vi "UTL_Generar Reporte.vi"(8 "Error in":errorcluster, 10 "Data":dbl[][](array[numeric]), 11 "Results Path":path) -> (0 "Error out":errorcluster, 3 "Tabla de Datos":string[][](array[string]))   [LabVIEW 2019]
uses:
  Variable global de carga.vi
  <vilib>/Utility/file.llb/Read Delimited Spreadsheet (string).vi
  <vilib>/Utility/file.llb/Write Delimited Spreadsheet (string).vi
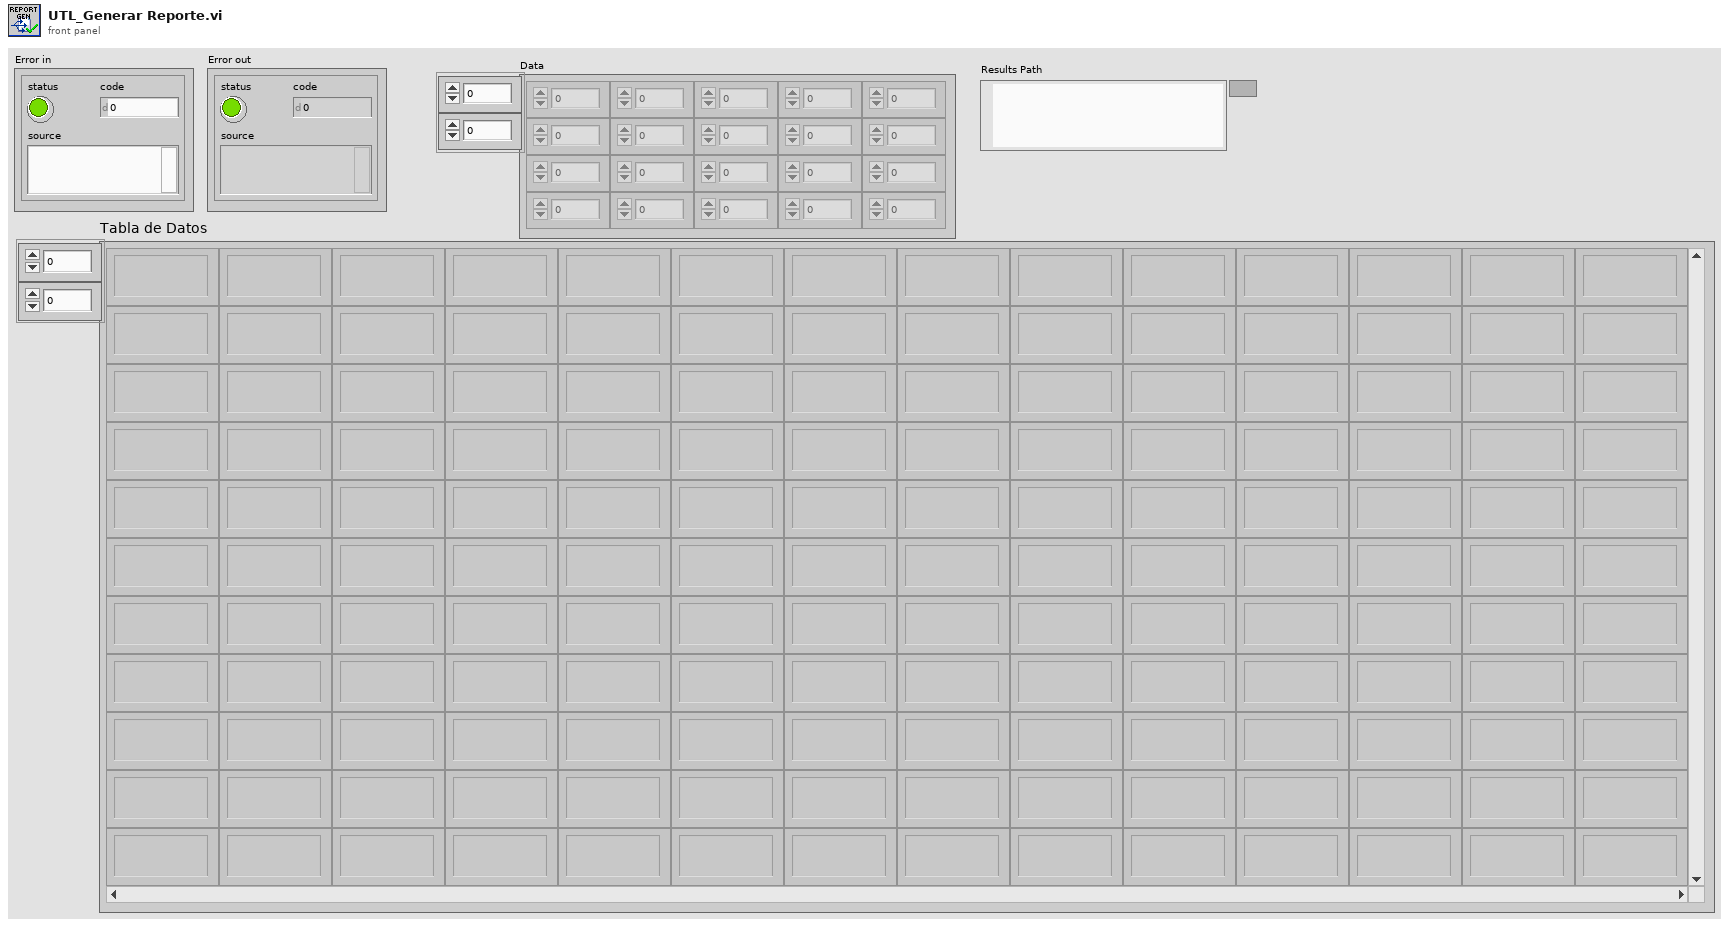
[diagram p1: front panel]
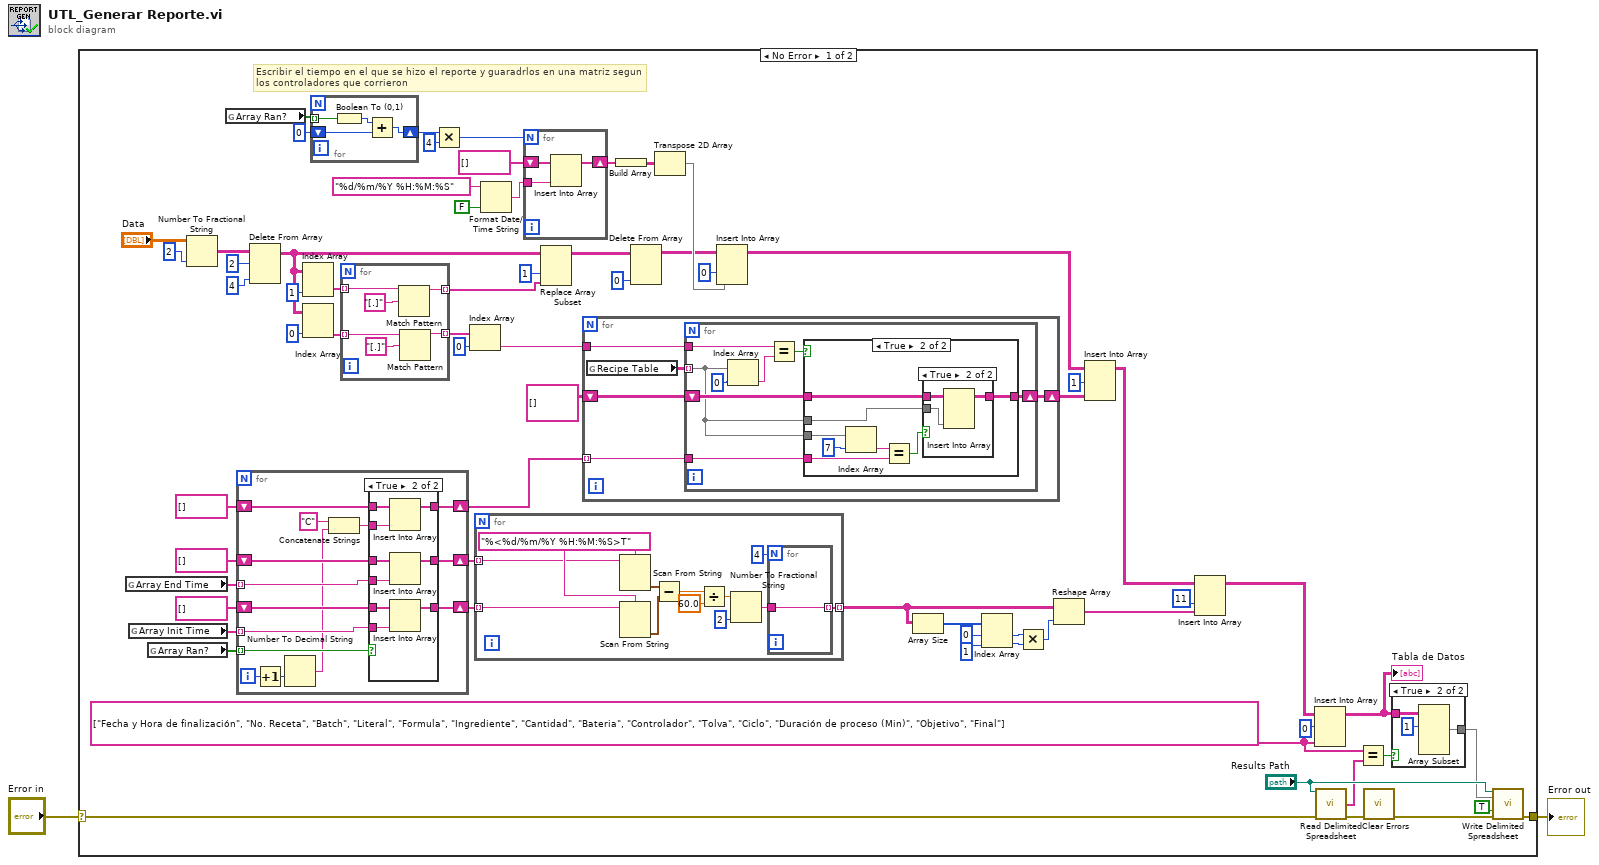
[diagram p0: block diagram]
diagram:
  n1 = case shown="No Error" "Error in" {
    selector: "Error in" -> [w53 w152]
    tunnel: [w63 w152] -> w1
    frame No Error {
      w16 = string[] ["Fecha y Hora de finalización", "No. Receta", "Batch", "Literal", "Formula", "Ingrediente", "Cantidad", "Bateria", "Controlador", "Tolva", "Ciclo", "Duración de proceso (Min)", "Objetivo", "Final"]
      # "Escribir el tiempo en el que se hizo el reporte y guaradrlos en una matriz segun los controladores que corrieron"
      n2 = global read "Variable global de carga.vi" "Array End Time"() -> (w21:string[])
      n3 = global read "Variable global de carga.vi" "Array Init Time"() -> (w22:string[])
      n4 = global read "Variable global de carga.vi" "Array Ran?"() -> (w23:bool[])
      n5 = Number To Fractional String(number="Data", precision (6)=i16 2) -> (F-format string=w11:string[][])  [unwired: 2 in]
      n6 = global read "Variable global de carga.vi" "Array Ran?"() -> (w28:bool[])
      n7 = for {
        tunnel: w23 -> [w96] mode=indexing
        shift-right: [w94] -> w46
        shift-left: string[] [] -> [w95]
        shift-right: [w92] -> w20
        shift-left: string[] [] -> [w93]
        shift-right: [w91] -> w19
        shift-left: string[] [] -> [w90]
        tunnel: w22 -> [w89] mode=indexing
        tunnel: w21 -> [w88] mode=indexing
        i -> [w87]
        n8 = Increment(x=w87) -> (x+1=w86:i32)
        n9 = Number To Decimal String(number=w86) -> (decimal integer string=w85:string)  [unwired: 1 in]
        n10 = Concatenate Strings("C" ("string"), w85) -> (w83:string)
        n11 = case shown="True" w96 {
          tunnel: w95 -> [w99 w108]
          tunnel: [w99 w107] -> w94
          tunnel: w93 -> [w98 w106]
          tunnel: [w98 w105] -> w92
          tunnel: w90 -> [w97 w103]
          tunnel: [w97 w104] -> w91
          tunnel: w89 -> [_ w102]
          tunnel: w88 -> [_ w101]
          tunnel: w83 -> [_ w100]
          frame False {
          }
          frame True {
            n12 = Insert Into Array(array=w108, new element=w100) -> (w107:string[])  [unwired: 1 in]
            n13 = Insert Into Array(array=w106, new element=w101) -> (w105:string[])  [unwired: 1 in]
            n14 = Insert Into Array(array=w103, new element=w102) -> (w104:string[])  [unwired: 1 in]
          }
        }
      }
      n15 = Delete From Array(array=w11, length=2, index (col)=4 ("disabled index (col)")) -> (array with subset deleted=w7:string[][])  [unwired: 1 in, 1 out]
      n16 = Index Array(array=w7, index (col)=1 ("disabled index (col)")) -> (element=w8:string[])  [unwired: 1 in]
      n17 = Index Array(array=w7, index (col)=0 ("disabled index (col)")) -> (element=w61:string[])  [unwired: 1 in]
      n18 = for {
        tunnel: w28 -> [w112] mode=indexing
        shift-right: [w109] -> w29
        shift-left: 0 -> [w110]
        n19 = Boolean To (0,1)(Boolean=w112) -> (0, 1=w111:i16)
        n20 = Add(x=w111, y=w110) -> (x+y=w109:i32)
      }
      n21 = for {
        tunnel: w61 -> [w150] mode=indexing
        tunnel: [w149] -> w35 mode=indexing
        tunnel: w8 -> [w147] mode=indexing
        tunnel: [w146] -> w4 mode=indexing
        n22 = Match Pattern(string=w147, regular expression="[.]") -> (before substring=w146:string)  [unwired: 1 in, 3 out]
        n23 = Match Pattern(string=w150, regular expression="[.]") -> (before substring=w149:string)  [unwired: 1 in, 3 out]
      }
      n24 = Multiply(x=w29, y=i16 4) -> (x*y=w27:i32)
      n25 = Index Array(array=w35, index=0) -> (element=w59:string)
      n26 = for {
        tunnel: w20 -> [w71] mode=indexing
        tunnel: w19 -> [w72] mode=indexing
        tunnel: [w70] -> w18 mode=indexing
        w73 = "%<%d/%m/%Y %H:%M:%S>T" ("format string")
        n27 = Scan From String(format string=w73, input string=w71) -> (output 1=w77:timestamp)  [unwired: 3 in, 3 out]
        n28 = Scan From String(format string=w73, input string=w72) -> (output 1=w78:timestamp)  [unwired: 3 in, 3 out]
        n29 = Subtract(x=w77, y=w78) -> (x-y=w80:dbl)
        n30 = Divide(x=w80, y=60.0) -> (x/y=w79:dbl)
        n31 = Number To Fractional String(number=w79, precision (6)=i16 2) -> (F-format string=w81:string)  [unwired: 2 in]
        n32 = for {
          N: 4 -> [_]
          tunnel: w81 -> [w82]
          tunnel: [w82] -> w70 mode=indexing
        }
      }
      n33 = Format Date/Time String(time format string (%c)="%d/%m/%Y %H:%M:%S", UTC format=FALSE) -> (date/time string=w47:string)  [unwired: 1 in]
      n34 = for {
        N: w27 -> [_]
        tunnel: w47 -> [w141]
        shift-right: [w139] -> w48
        shift-left: string[] [] -> [w140]
        n35 = Insert Into Array(array=w140, new element=w141) -> (w139:string[])  [unwired: 1 in]
      }
      n36 = Replace Array Subset(array=w7, new element=w4, index (col)=1 ("disabled index (col)")) -> (w6:string[][])  [unwired: 1 in]
      n37 = for {
        tunnel: w59 -> [w117]
        tunnel: w46 -> [w116] mode=indexing
        shift-right: [w114] -> w57
        shift-left: string[][] [] -> [w115]
        n38 = global read "Variable global de carga.vi" "Recipe Table"() -> (w113:string[][])
        n39 = for {
          tunnel: w113 -> [w120] mode=indexing
          tunnel: w117 -> [w119]
          tunnel: w116 -> [w123]
          shift-right: [w121] -> w114
          shift-left: w115 -> [w122]
          n40 = Index Array(array=w120, index=0) -> (element=w118:string)
          n41 = Equal?(x=w119, y=w118) -> (x = y?=w124:bool)
          n42 = case shown="True" w124 {
            tunnel: w120 -> [_ w134]
            tunnel: w123 -> [_ w131]
            tunnel: [w126 w128] -> w121
            tunnel: w122 -> [w126 w129]
            tunnel: w120 -> [_ w127]
            frame False {
            }
            frame True {
              n43 = Index Array(array=w134, index=7) -> (element=w132:string)
              n44 = Equal?(x=w132, y=w131) -> (x = y?=w130:bool)
              n45 = case shown="True" w130 {
                tunnel: w129 -> [w135 w138]
                tunnel: [w135 w137] -> w128
                tunnel: w127 -> [_ w136]
                frame False {
                }
                frame True {
                  n46 = Insert Into Array(array=w138, new element=w136) -> (w137:string[][])  [unwired: 2 in]
                }
              }
            }
          }
        }
      }
      n47 = Build Array(w48) -> (w66:string[][])
      n48 = Delete From Array(array=w6, index (col)=0 ("disabled index (col)")) -> (array with subset deleted=w34:string[][])  [unwired: 2 in, 1 out]
      n49 = Transpose 2D Array(2D array=w66) -> (transposed array=w65:string[][])
      n50 = Insert Into Array(array=w34, index (col)=0 ("disabled index (col)"), new element=w65) -> (w10:string[][])  [unwired: 1 in]
      n51 = Array Size(array=w18) -> (size(s)=w43:i32[])
      n52 = Index Array(array=w43, index #1=0 ("index"), index #2=1 ("index")) -> (element #1=w40:i32, element #2=w39:i32)
      n53 = Multiply(x=w40, y=w39) -> (x*y=w38:i32)
      n54 = Reshape Array(w18, w38) -> (w37:string[])
      n55 = Insert Into Array(array=w10, index (col)=1, new element=w57) -> (w17:string[][])  [unwired: 1 in]
      n56 = Insert Into Array(array=w17, index (col)=11 ("disabled index (col)"), new element=w37) -> (w55:string[][])  [unwired: 1 in]
      n57 = Insert Into Array(array=w55, index (row)=0, new element=w16) -> (w36:string[][])  [unwired: 1 in]
      "Tabla de Datos" <- w36
      n58 = call-poly <vilib>:"Read Delimited Spreadsheet.vi"("file path (dialog if empty)"="Results Path", "error in (no error)"=w53) -> ("first row"=w15:string[], "error out"=w50:errorcluster)  [unwired: 8 in, 4 out]
      n59 = Equal?(x=w16, y=w15) -> (x = y?=w62:bool)
      n60 = call <vilib>:"Clear Errors.vi"("error in (no error)"=w50) -> ("error out"=w14:errorcluster)  [unwired: 5 in, 1 out]
      n61 = case shown="True" w62 {
        tunnel: w36 -> [w142 w145]
        tunnel: [w142 w144] -> w32
        frame False {
        }
        frame True {
          n62 = Array Subset(array=w145, index (row)=1 ("index")) -> (w144:string[][])  [unwired: 3 in]
        }
      }
      n63 = call-poly <vilib>:"Write Delimited Spreadsheet.vi"("file path (dialog if empty)"="Results Path", "2D data"=w32, "append to file? (new file:F)"=TRUE, "error in (no error)"=w14) -> ("error out"=w63:errorcluster)  [unwired: 10 in, 1 out]
    }
    frame Error {
    }
  }
  "Error out" <- w1
